vi "Channel Mng Performance Test.vi"() -> ()   [LabVIEW 2021]
uses:
  CIFChannels/Typedef/Direction.ctl
  CIF_NIChn/Double/CIF_NIChn_Double.lvclass
  D:/dev/Packages/Channel_Manager/src/CIFChannels/CIFChannels.lvclass
  <vilib>/Platform/TimedLoop/XDataNode/timing_clust.ctl
  <vilib>/Platform/TimedLoop/XDataNode/nitl_modes.ctl
  <vilib>/Platform/TimedLoop/XDataNode/wakeup.ctl
  CIFChannelMng.lvclass
  CIFChannels/CIFChannels.lvclass/CIFChannels.ctl
  CIFChannelMng.lvclass/CIFChannelMng.ctl
  7d13c5b7-0b44-4ab4-8a6c-0bcd63b70b59.vi
  c0ba1b46-a5a0-42bd-afb3-2f6832d2a88c.vi
  6a1b8880-d4c2-444f-a4b2-811244e6db06.vi
  10e1b524-69ef-478e-ae98-36060d5eb0d6.vi
  332321e3-b478-4438-b8ac-43cf378b23bb.vi
  <vilib>/CIFChannels/SubVIs/Add Error.vi
  7d13c5b7-0b44-4ab4-8a6c-0bcd63b70b59.vi/c28b0ead-42ad-4072-80a2-aca7f2bd7ce3.vi
  <vilib>/CIFChannels/SubVIs/CIFServices Fill In Error Info Ex.vi
  <vilib>/CIFChannels/SubVIs/Get dll Path.vi
  c0ba1b46-a5a0-42bd-afb3-2f6832d2a88c.vi/4bc1c15b-36ab-481f-b8dd-c64075ce723a.vi
  c0ba1b46-a5a0-42bd-afb3-2f6832d2a88c.vi/d83cb72b-7713-41fc-a3d1-682de79cf574.vi
  6a1b8880-d4c2-444f-a4b2-811244e6db06.vi/c28b0ead-42ad-4072-80a2-aca7f2bd7ce3.vi
  10e1b524-69ef-478e-ae98-36060d5eb0d6.vi/c28b0ead-42ad-4072-80a2-aca7f2bd7ce3.vi
  10e1b524-69ef-478e-ae98-36060d5eb0d6.vi/219d0231-d98b-4193-b5cc-84f90e3c9091.vi
  332321e3-b478-4438-b8ac-43cf378b23bb.vi/c28b0ead-42ad-4072-80a2-aca7f2bd7ce3.vi
  332321e3-b478-4438-b8ac-43cf378b23bb.vi/219d0231-d98b-4193-b5cc-84f90e3c9091.vi
  ChannelCommon/Utilities/Add Error.vi
  CIFChannels/Accessors/Read Name.vi
  CIFChannels/Accessors/Read Custom Config Data.vi
  CIFChannels/Accessors/Read Type.vi
  CIFChannels/Accessors/Read Direction.vi
  Utilities/Get Channel Index by Name.vi
  CIFChannels/Accessors/Read Channel State.vi
  Utilities/Remove Channel by Index.vi
  <vilib>/CIFChannels/SubVIs/Append Error Location.vi
  <vilib>/CIF Foundation/CIF Utilities/Errors/Append Error Location.vi
  CIFChannels/Accessors/Write Channel State.vi
  <vilib>/Platform/TimedLoop/XDataNode/XDataNode.xnode
  CIFChannels/CIFChannels.lvclass
  <vilib>/Platform/TimedLoop/XDataNode/XDNodeRunTimeDep.lvlib
  <vilib>/CIFChannels/CIFChannelCore.lvlib
panel:
  out "avg dbl channel":dbl
  out "max dbl channel":dbl
  out "avg raw channel":dbl
  out "max raw channel":dbl
  out "pass":bool
  out "error out":errorcluster
  # "This test should be run on RT.  It stresses the communications by constantly creating resource contraints with the low priority sender and the high priority loop. On Windows the priority of the loops cannot be set."
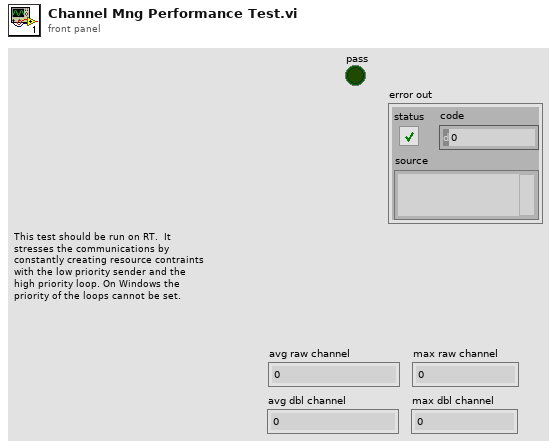
[diagram p1: front panel]
types:
  T1 = typedef "CIFChannels.lvclass/Direction.ctl" = enum16{"Publisher", "Subscriber"}
  T2 = typedef "XDNodeRunTimeDep.lvlib/timing_clust.ctl" = cluster{"Expected End [f-1]":u64, "Actual End [f-1]":u64, "Finished Late? [f-1]":bool, "Expected End [i-1]":u64, "Actual End [i-1]":u64, "Finished Late? [i-1]":bool, "Expected Start [i]":u64, "Actual Start [i]":u64, "Expected Start [f]":u64, "Actual Start [f]":u64, "Source Name":string, "Structure Name":string, "Period":i64, "Deadline":i64, "Offset":i64, "Start":i64, "Priority":i32, "Timeout":i32, "Mode":T3, "Wakeup Reason":T4, "Error":errorcluster, "Source Type":string, "Secondary Source Type":string, "Global End Time":u64, "Global Start Time":u64, "Frame Duration":u64, "Iteration Duration":u64, "Assigned CPU":i32, "I/O Scan Engine Mode":u32}
  T3 = typedef "XDNodeRunTimeDep.lvlib/nitl_modes.ctl" = enum32{"No Change", "Process missed periods, maintain original phase", "Discard missed periods, maintain original phase", "Process missed periods, ignore original phase", "Discard missed periods, ignore original phase"}
  T4 = typedef "XDNodeRunTimeDep.lvlib/wakeup.ctl" = enum32{"Normal", "Aborted", "Asynchronous wakeup", "Timing source error", "Timed loop error", "Timeout"}
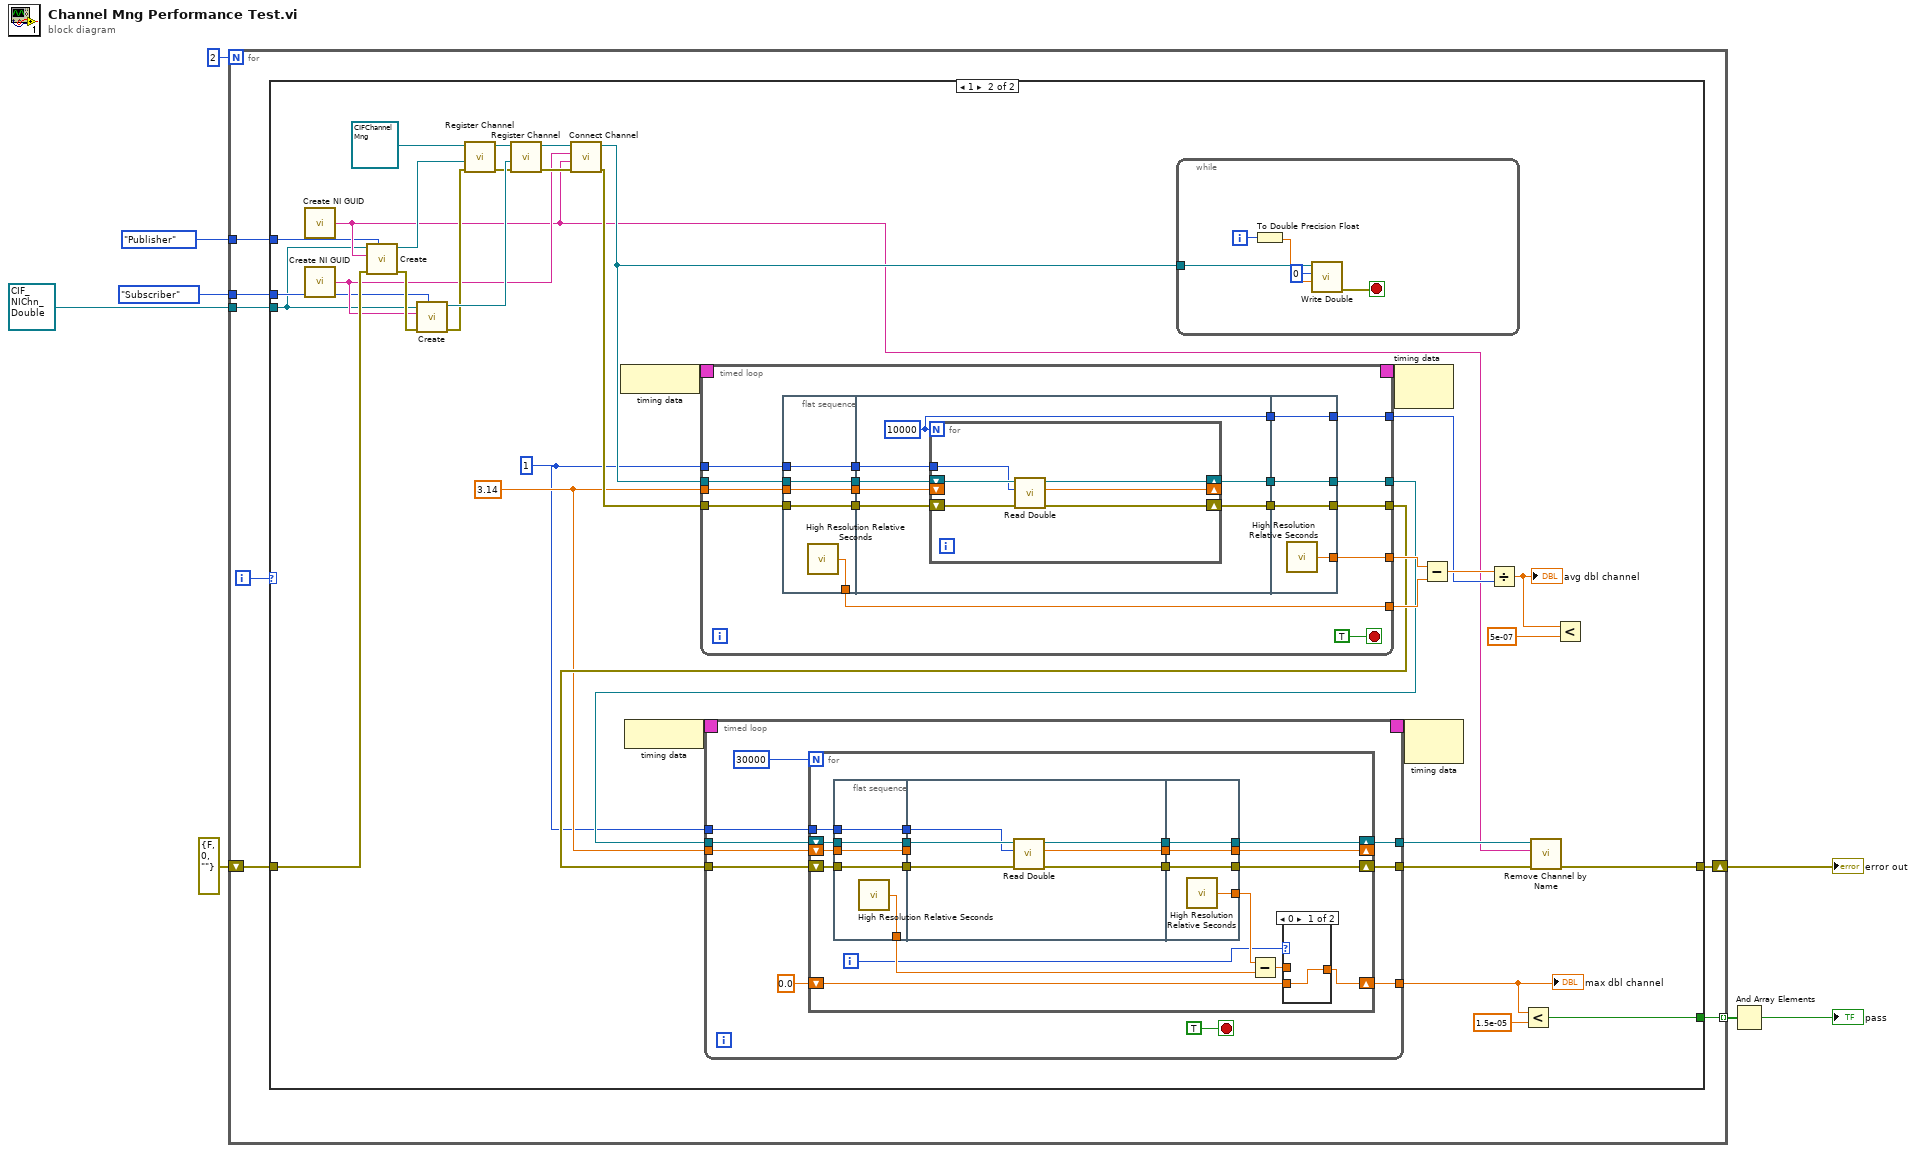
[diagram p0: block diagram]
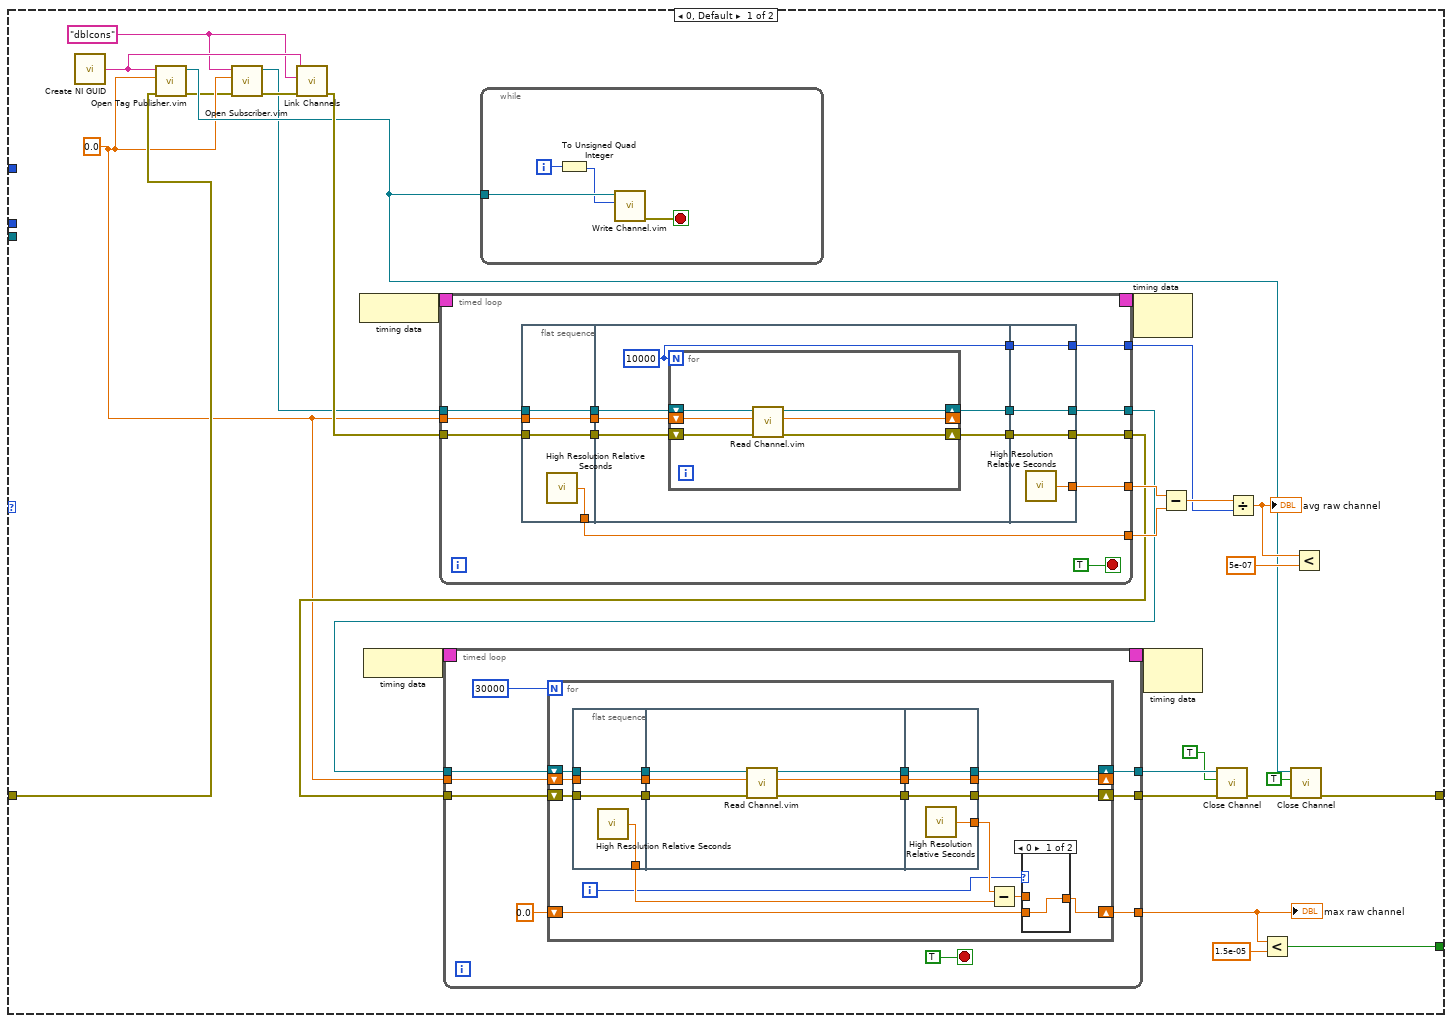
[diagram p2: hidden frame]
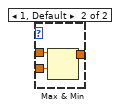
[diagram p3: hidden frame]
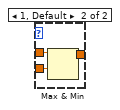
[diagram p4: hidden frame]
diagram:
  n1 = for {
    N: 2 -> [_]
    tunnel: [w15] -> w6 mode=indexing
    shift-right: [w14] -> w8
    shift-left: errorcluster {"status"=FALSE, "code"=0, "source"=""} ("error out") -> [w12]
    tunnel: Direction."Publisher" ("Direction") -> [w11]
    tunnel: Direction."Subscriber" ("Direction") -> [w10]
    tunnel: refnum<class "CIF_NIChn_Double.lvclass"> refnum ("CIFTag in") -> [w9]
    i -> [w13]
    n2 = case shown="1" w13 {
      tunnel: [w31 w160] -> w15
      tunnel: [w24 w143] -> w14
      tunnel: w12 -> [w29 w150]
      tunnel: w11 -> [_ w141]
      tunnel: w10 -> [_ w140]
      tunnel: w9 -> [_ w139]
      frame 0, Default {
        w18 = "dblcons" ("Channel Name")
        w20 = 0.0
        n3 = call <vilib>:"Create NI GUID.vi"() -> ("NI GUID"=w22:string)
        n4 = call "Open Tag Publisher.vim"("error in"=w29, "Input Type"=w20, "Channel Name"=w22) -> ("error out"=w19:errorcluster, "CIF Channel"=w23:refnum<k21>)  [unwired: 7 in]
        n5 = call "Open Subscriber.vim"("error in"=w19, "Input Type"=w20, "Channel Name"=w18) -> ("error out"=w17:errorcluster, "CIF Channel"=w16:refnum<k21>)  [unwired: 7 in]
        n6 = call <vilib>:"Link Channels.vi"("error in"=w17, "Consumer Channel Name"=w18, "Producer Channel Name"=w22) -> ("error out"=w30:errorcluster)  [unwired: 8 in]
        n7 = node-c288() -> (w45:T2)
        n8 = node-c288() -> (w43:T2)
        n9 = timed-loop {
          timing: w45 -> [_]
          timing-out: [_] -> w44
          tunnel: w16 -> [w113]
          tunnel: w30 -> [w112]
          tunnel: [w108] -> w37
          tunnel: [w106] -> w36
          tunnel: [w104] -> w41
          tunnel: [w103] -> w40
          tunnel: [w102] -> w38
          tunnel: w20 -> [w100]
          stop <- TRUE stop-if-true
          n10 = flat-sequence {
            tunnel: w112 -> [w116]
            tunnel: w113 -> [w117]
            tunnel: [w117] -> w110
            tunnel: [w116] -> w109
            tunnel: [w115] -> w103
            tunnel: w100 -> [w114]
            tunnel: [w114] -> w99
            tunnel: w110 -> [w123]
            tunnel: w109 -> [w122]
            tunnel: [w121] -> w107
            tunnel: [w120] -> w105
            tunnel: [w119] -> w101
            tunnel: w99 -> [w118]
            tunnel: [w133] -> w108
            tunnel: w107 -> [w133]
            tunnel: [w132] -> w106
            tunnel: w105 -> [w132]
            tunnel: [w131] -> w104
            tunnel: [w130] -> w102
            tunnel: w101 -> [w130]
            frame #0 {
              n11 = call <vilib>:"High Resolution Relative Seconds.vi"() -> ("relative seconds"=w115:dbl)
            }
            frame #1 {
              w119 = 10000
              n12 = for {
                N: w119 -> [_]
                shift-right: [w126] -> w121
                shift-left: w123 -> [w129]
                shift-right: [w125] -> w120
                shift-left: w122 -> [w124]
                shift-right: [w127] -> _
                shift-left: w118 -> [w128]
                n13 = call "Read Channel.vim"("error in"=w124, "Data in"=w128, "CIF Channel in"=w129) -> ("error out"=w125:errorcluster, "Data out"=w127:dbl, "CIF Channel out"=w126:refnum<k21>)  [unwired: 5 in, 1 out]
              }
            }
            frame #2 {
              n14 = call <vilib>:"High Resolution Relative Seconds.vi"() -> ("relative seconds"=w131:dbl)
            }
          }
        }
        n15 = timed-loop {
          timing: w43 -> [_]
          timing-out: [_] -> w42
          tunnel: w37 -> [w58]
          tunnel: w36 -> [w57]
          tunnel: [w55] -> w27
          tunnel: [w54] -> w28
          tunnel: w20 -> [w53]
          tunnel: [w50] -> w33
          stop <- TRUE stop-if-true
          n16 = for {
            N: 30000 -> [_]
            shift-right: [w70] -> w55
            shift-left: w58 -> [w72]
            shift-right: [w69] -> w54
            shift-left: w57 -> [w71]
            shift-right: [w63] -> w50
            shift-left: 0.0 -> [w64]
            shift-right: [w62] -> _
            shift-left: w53 -> [w68]
            i -> [w60]
            n17 = flat-sequence {
              tunnel: w71 -> [w83]
              tunnel: w72 -> [w84]
              tunnel: [w84] -> w76
              tunnel: [w83] -> w75
              tunnel: [w82] -> w66
              tunnel: w68 -> [w81]
              tunnel: [w81] -> w74
              tunnel: w76 -> [w90]
              tunnel: w75 -> [w86]
              tunnel: [w89] -> w73
              tunnel: w74 -> [w88]
              tunnel: [w87] -> w61
              tunnel: [w85] -> w59
              tunnel: [w94] -> w70
              tunnel: w73 -> [w94]
              tunnel: [w93] -> w69
              tunnel: [w92] -> w67
              tunnel: [w91] -> w62
              tunnel: w61 -> [w91]
              tunnel: w59 -> [w93]
              frame #0 {
                n18 = call <vilib>:"High Resolution Relative Seconds.vi"() -> ("relative seconds"=w82:dbl)
              }
              frame #1 {
                n19 = call "Read Channel.vim"("error in"=w86, "Data in"=w88, "CIF Channel in"=w90) -> ("error out"=w85:errorcluster, "Data out"=w87:dbl, "CIF Channel out"=w89:refnum<k21>)  [unwired: 5 in, 1 out]
              }
              frame #2 {
                n20 = call <vilib>:"High Resolution Relative Seconds.vi"() -> ("relative seconds"=w92:dbl)
              }
            }
            n21 = Subtract(x=w67, y=w66) -> (x-y=w65:dbl)
            n22 = case shown="0" w60 {
              tunnel: w65 -> [_ w80]
              tunnel: w64 -> [w77 w79]
              tunnel: [w77 w78] -> w63
              frame 0 {
              }
              frame 1, Default {
                n23 = Max & Min(x=w80, y=w79) -> (max(x,y)=w78:dbl)  [unwired: 1 out]
              }
            }
          }
        }
        "max raw channel" <- w33
        n24 = while {
          tunnel: w23 -> [w48]
          i -> [w49]
          stop <- w46 stop-if-true
          n25 = To Unsigned Quad Integer(1:w49) -> (0:w47:u64)
          n26 = call "Write Channel.vim"("Data in"=w47, "CIF Channel in"=w48) -> ("error out"=w46:errorcluster)  [unwired: 6 in, 3 out]
        }
        n27 = node-c288(w44) -> ()  [unwired: 1 out]
        n28 = node-c288(w42) -> ()  [unwired: 1 out]
        n29 = Subtract(x=w41, y=w40) -> (x-y=w39:dbl)
        n30 = call <vilib>:"Close Channel.vi"("error in"=w28, "Force Destroy? (F)"=TRUE, "CIF Channel"=w27) -> ("error out"=w26:errorcluster)  [unwired: 8 in]
        n31 = Divide(x=w39, y=w38) -> (x/y=w35:dbl)
        "avg raw channel" <- w35
        n32 = Less?(x=w33, y=1.5e-05) -> (x < y?=w31:bool)
        n33 = call <vilib>:"Close Channel.vi"("error in"=w26, "Force Destroy? (F)"=TRUE, "CIF Channel"=w23) -> ("error out"=w24:errorcluster)  [unwired: 8 in]
        n34 = Less?(x=w35, y=5e-07) -> ()  [unwired: 1 out]
      }
      frame 1 {
        w138 = 1 ("Channel Index")
        w147 = 3.14 ("Default Value")
        n35 = call <vilib>:"Create NI GUID.vi"() -> ("NI GUID"=w142:string)
        n36 = call <vilib>:"Create NI GUID.vi"() -> ("NI GUID"=w146:string)
        n37 = call-dynamic "Create.vi"("Direction"=w141, "error in (no error)"=w150, "Name"=w142, "CIFTag in"=w139) -> ("error out"=w155:errorcluster, "CIFTag out"=w154:refnum<class "CIF_NIChn_Double.lvclass">)  [unwired: 6 in]
        n38 = call-dynamic "Create.vi"("Direction"=w140, "error in (no error)"=w155, "Name"=w146, "CIFTag in"=w139) -> ("error out"=w156:errorcluster, "CIFTag out"=w159:refnum<class "CIF_NIChn_Double.lvclass">)  [unwired: 6 in]
        n39 = call "Register Channel.vi"("error in (no error)"=w156, "Channel"=w154, "CIFChannelMng in"=refnum<class "CIFChannelMng.lvclass"> refnum) -> ("error out"=w153:errorcluster, "CIFChannelMng out"=w152:refnum<class "CIFChannelMng.lvclass">)  [unwired: 7 in]
        n40 = call "Register Channel.vi"("error in (no error)"=w153, "Channel"=w159, "CIFChannelMng in"=w152) -> ("error out"=w158:errorcluster, "CIFChannelMng out"=w157:refnum<class "CIFChannelMng.lvclass">)  [unwired: 7 in]
        n41 = call "Connect Channel.vi"("error in (no error)"=w158, "Publisher Name"=w142, "Subscriber Name"=w146, "CIFChannelMng in"=w157) -> ("error out"=w149:errorcluster, "CIFChannelMng out"=w148:refnum<class "CIFChannelMng.lvclass">)  [unwired: 6 in]
        n42 = node-c288() -> (w174:T2)
        n43 = node-c288() -> (w172:T2)
        n44 = timed-loop {
          timing: w174 -> [_]
          timing-out: [_] -> w173
          tunnel: w148 -> [w249]
          tunnel: w149 -> [w248]
          tunnel: [w244] -> w166
          tunnel: [w242] -> w165
          tunnel: [w240] -> w170
          tunnel: [w239] -> w169
          tunnel: [w238] -> w167
          tunnel: w147 -> [w236]
          tunnel: w138 -> [w234]
          stop <- TRUE stop-if-true
          n45 = flat-sequence {
            tunnel: w248 -> [w253]
            tunnel: w249 -> [w254]
            tunnel: [w254] -> w246
            tunnel: [w253] -> w245
            tunnel: [w252] -> w239
            tunnel: w236 -> [w251]
            tunnel: [w251] -> w235
            tunnel: w234 -> [w250]
            tunnel: [w250] -> w233
            tunnel: w246 -> [w261]
            tunnel: w245 -> [w260]
            tunnel: [w259] -> w243
            tunnel: [w258] -> w241
            tunnel: [w257] -> w237
            tunnel: w235 -> [w256]
            tunnel: w233 -> [w255]
            tunnel: [w271] -> w244
            tunnel: w243 -> [w271]
            tunnel: [w270] -> w242
            tunnel: w241 -> [w270]
            tunnel: [w269] -> w240
            tunnel: [w268] -> w238
            tunnel: w237 -> [w268]
            frame #0 {
              n46 = call <vilib>:"High Resolution Relative Seconds.vi"() -> ("relative seconds"=w252:dbl)
            }
            frame #1 {
              w257 = 10000
              n47 = for {
                N: w257 -> [_]
                shift-right: [w266] -> w259
                shift-left: w261 -> [w267]
                shift-right: [w265] -> w258
                shift-left: w260 -> [w264]
                shift-right: [w263] -> _
                shift-left: w256 -> [_]
                tunnel: w255 -> [w262]
                n48 = call "Read Double.vi"("error in (no error)"=w264, "Channel Index"=w262, "CIFChannelMng in"=w267) -> ("error out"=w265:errorcluster, "Data"=w263:dbl, "CIFChannelMng out"=w266:refnum<class "CIFChannelMng.lvclass">)  [unwired: 5 in, 1 out]
              }
            }
            frame #2 {
              n49 = call <vilib>:"High Resolution Relative Seconds.vi"() -> ("relative seconds"=w269:dbl)
            }
          }
        }
        n50 = timed-loop {
          timing: w172 -> [_]
          timing-out: [_] -> w171
          tunnel: w166 -> [w189]
          tunnel: w165 -> [w188]
          tunnel: [w186] -> w145
          tunnel: [w185] -> w144
          tunnel: w147 -> [w184]
          tunnel: [w181] -> w162
          tunnel: w138 -> [w180]
          stop <- TRUE stop-if-true
          n51 = for {
            N: 30000 -> [_]
            shift-right: [w203] -> w186
            shift-left: w189 -> [w205]
            shift-right: [w202] -> w185
            shift-left: w188 -> [w204]
            shift-right: [w196] -> w181
            shift-left: 0.0 -> [w197]
            shift-right: [w195] -> _
            shift-left: w184 -> [w201]
            tunnel: w180 -> [w191]
            i -> [w193]
            n52 = flat-sequence {
              tunnel: w204 -> [w217]
              tunnel: w205 -> [w218]
              tunnel: [w218] -> w209
              tunnel: [w217] -> w208
              tunnel: [w216] -> w199
              tunnel: w201 -> [w215]
              tunnel: [w215] -> w207
              tunnel: w191 -> [w214]
              tunnel: [w214] -> w190
              tunnel: w209 -> [w223]
              tunnel: w208 -> [w224]
              tunnel: [w222] -> w206
              tunnel: w207 -> [_]
              tunnel: [w220] -> w194
              tunnel: [w221] -> w192
              tunnel: w190 -> [w219]
              tunnel: [w228] -> w203
              tunnel: w206 -> [w228]
              tunnel: [w227] -> w202
              tunnel: [w226] -> w200
              tunnel: [w225] -> w195
              tunnel: w194 -> [w225]
              tunnel: w192 -> [w227]
              frame #0 {
                n53 = call <vilib>:"High Resolution Relative Seconds.vi"() -> ("relative seconds"=w216:dbl)
              }
              frame #1 {
                n54 = call "Read Double.vi"("error in (no error)"=w224, "Channel Index"=w219, "CIFChannelMng in"=w223) -> ("error out"=w221:errorcluster, "Data"=w220:dbl, "CIFChannelMng out"=w222:refnum<class "CIFChannelMng.lvclass">)  [unwired: 5 in, 1 out]
              }
              frame #2 {
                n55 = call <vilib>:"High Resolution Relative Seconds.vi"() -> ("relative seconds"=w226:dbl)
              }
            }
            n56 = Subtract(x=w200, y=w199) -> (x-y=w198:dbl)
            n57 = case shown="0" w193 {
              tunnel: w198 -> [_ w213]
              tunnel: w197 -> [w210 w212]
              tunnel: [w210 w211] -> w196
              frame 0 {
              }
              frame 1, Default {
                n58 = Max & Min(x=w213, y=w212) -> (max(x,y)=w211:dbl)  [unwired: 1 out]
              }
            }
          }
        }
        "max dbl channel" <- w162
        n59 = while {
          tunnel: w148 -> [w178]
          i -> [w179]
          stop <- w176 stop-if-true
          n60 = To Double Precision Float(number=w179) -> (double precision float=w177:dbl)
          n61 = call "Write Double.vi"("Data"=w177, "Channel Index"=0, "CIFChannelMng in"=w178) -> ("error out"=w176:errorcluster)  [unwired: 6 in, 2 out]
        }
        n62 = node-c288(w173) -> ()  [unwired: 1 out]
        n63 = node-c288(w171) -> ()  [unwired: 1 out]
        n64 = Subtract(x=w170, y=w169) -> (x-y=w168:dbl)
        n65 = Divide(x=w168, y=w167) -> (x/y=w164:dbl)
        "avg dbl channel" <- w164
        n66 = Less?(x=w162, y=1.5e-05) -> (x < y?=w160:bool)
        n67 = call "Remove Channel by Name.vi"("error in (no error)"=w144, "Channel Name"=w142, "CIFChannelMng in"=w145) -> ("error out"=w143:errorcluster)  [unwired: 7 in, 1 out]
        n68 = Less?(x=w164, y=5e-07) -> ()  [unwired: 1 out]
      }
    }
  }
  "error out" <- w8
  n69 = And Array Elements(Boolean array=w6) -> (logical AND=→"pass":bool)
